vi "Read Props.vi"(8 "error in (no error)":errorcluster, 11 "DblNumericStatusEditorPanel in":refnum<class "DblNumericStatusEditorPanel.lvclass">) -> (0 "error out":errorcluster, 2 "Props":T1, 3 "DblNumericStatusEditorPanel out":refnum<class "DblNumericStatusEditorPanel.lvclass">)   [LabVIEW 2020, in "VolatusGUIControls.lvlib" / "DblNumericStatusEditorPanel.lvclass"]
uses:
  DblNumericStatusEditorPanel.lvclass
  DblNumericStatusEditorPanel.lvclass/DblNumericStatusEditorPanel.ctl
  VolatusGUIControls.lvlib
  e6f2d51f-dfc6-461f-bfa0-5a7a131bf987.vi
  JSON Props.ctl
  VolatusGUIEditorCore/Label Props.ctl
  VolatusGUIEditorCore/VolatusGUIEditorCore.lvlib
  VolatusGUIEditorCore/Position Props.ctl
  VolatusGUIEditorCore/Numeric Text Props.ctl
  Props.ctl
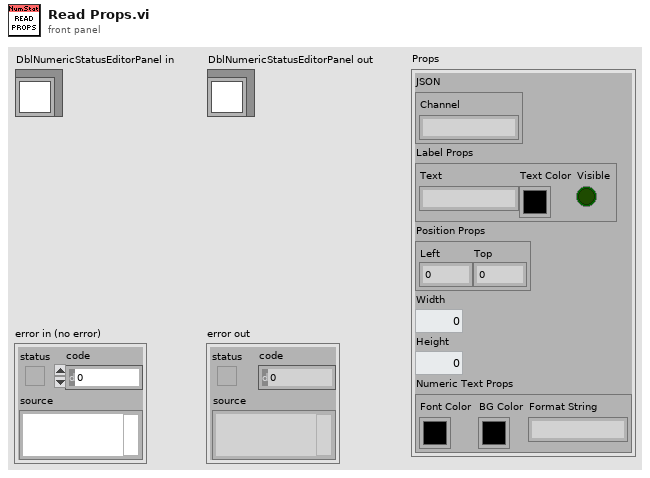
[diagram p1: front panel]
types:
  T1 = typedef "VolatusGUIControls.lvlib/DblNumericStatusEditorPanel.lvclass/Props.ctl" = cluster{"JSON":T2, "Label Props":T3, "Position Props":T4, "Width":u16, "Height":u16, "Numeric Text Props":T5}
  T2 = typedef "VolatusGUIControls.lvlib/DblNumericStatusEditorPanel.lvclass/JSON Props.ctl" = cluster{"Channel":string}
  T3 = typedef "VolatusGUIEditorCore.lvlib/Label Props.ctl" = cluster{"Text":string, "Text Color":u32, "Visible":bool}
  T4 = typedef "VolatusGUIEditorCore.lvlib/Position Props.ctl" = cluster{"Left":i32, "Top":i32}
  T5 = typedef "VolatusGUIEditorCore.lvlib/Numeric Text Props.ctl" = cluster{"Font Color":u32, "BG Color":u32, "Format String":string}
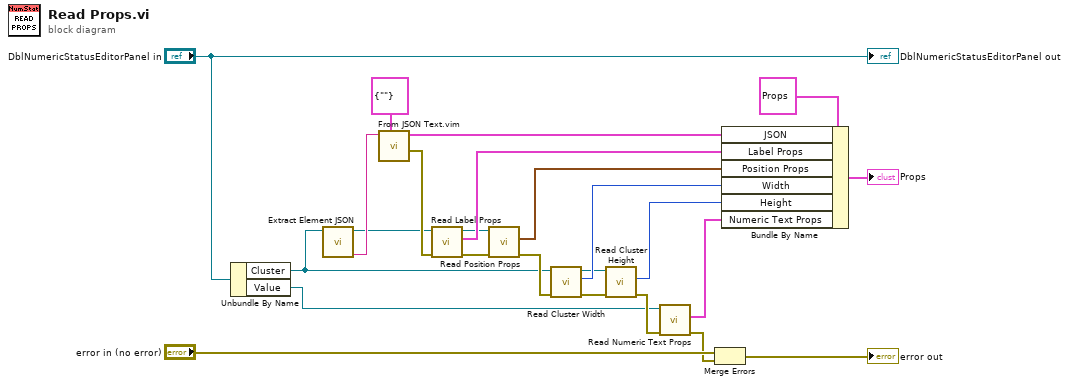
[diagram p0: block diagram]
diagram:
  n1 = Unbundle By Name("DblNumericStatusEditorPanel in") -> ("Cluster"=w10:refnum<vi>, "Value"=w4:refnum<vi>)
  n2 = call "Extract Element JSON.vi"("Ctl Refnum in"=w10) -> ("JSON"=w22:string, "Ctl Refnum"=w16:refnum<vi>)  [unwired: 7 in, 2 out]
  n3 = call "From JSON Text.vim"("Data Type and Default Value"=T2 {"Channel"=""} ("JSON"), "JSON"=w22) -> ("error out"=w17:errorcluster, "Data out"=w18:T2)  [unwired: 8 in]
  n4 = call "Read Label Props.vi"("error in (no error)"=w17, "Ctl Refnum in"=w16) -> ("error out"=w14:errorcluster, "Label Props"=w15:T3, "Ctl Refnum"=w13:refnum<vi>)  [unwired: 7 in]
  n5 = call "Read Position Props.vi"("error in (no error)"=w14, "Ctl Refnum in"=w13) -> ("error out"=w11:errorcluster, "Position Props"=w12:T4)  [unwired: 7 in, 1 out]
  n6 = call "Read Cluster Width.vi"("error in (no error)"=w11, "Cluster in"=w10) -> ("error out"=w8:errorcluster, "Width"=w9:i32, "Cluster"=w7:refnum<vi>)  [unwired: 7 in]
  n7 = call "Read Cluster Height.vi"("error in (no error)"=w8, "Cluster in"=w7) -> ("error out"=w5:errorcluster, "Height"=w6:i32)  [unwired: 7 in, 1 out]
  n8 = call "Read Numeric Text Props.vi"("error in"=w5, "Control in"=w4) -> ("error out"=w1:errorcluster, "Numeric Text Props"=w3:T5)  [unwired: 7 in, 1 out]
  n9 = Merge Errors("error in (no error)", w1) -> (→"error out":errorcluster)
  n10 = Bundle By Name(cluster=T1 {"JSON"={"Channel"=""}, "Label Props"={"Text"="", "Text Color"=0, "Visible"=FALSE}, "Position Props"={"Left"=0, "Top"=0}, "Width"=0, "Height"=0, "Numeric Text Props"={"Font Color"=0, "BG Color"=0, "Format String"=""}} ("Props"), "JSON"=w18, "Label Props"=w15, "Position Props"=w12, "Width"=w9, "Height"=w6, "Numeric Text Props"=w3) -> (→"Props":T1)
  "DblNumericStatusEditorPanel out" <- "DblNumericStatusEditorPanel in"
